vi "pcfs_auxillary_loop.vi"(8 "error in (no error)":errorcluster, 11 "pcfs in":refnum<class "pcfs.lvclass">) -> (0 "error out":errorcluster, 3 "pcfs out":refnum<class "pcfs.lvclass">)   [LabVIEW 2015, in "pcfs.lvclass"]
uses:
  pcfs.lvclass
  pcfs.lvclass/pcfs.ctl
  Detector_Class/Picoquant/Picoquant_generic/picoquant_generic.lvclass
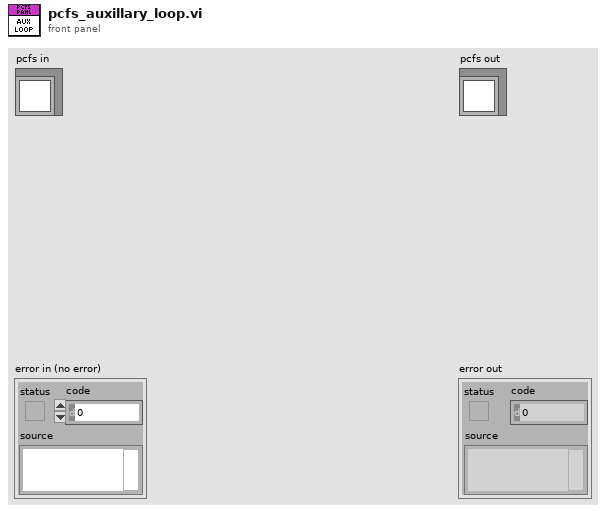
[diagram p1: front panel]
types:
  T1 = typedef "hydraharp_count_rates.ctl" = cluster{"channel_rates":i32[], "sync_rate":i32}
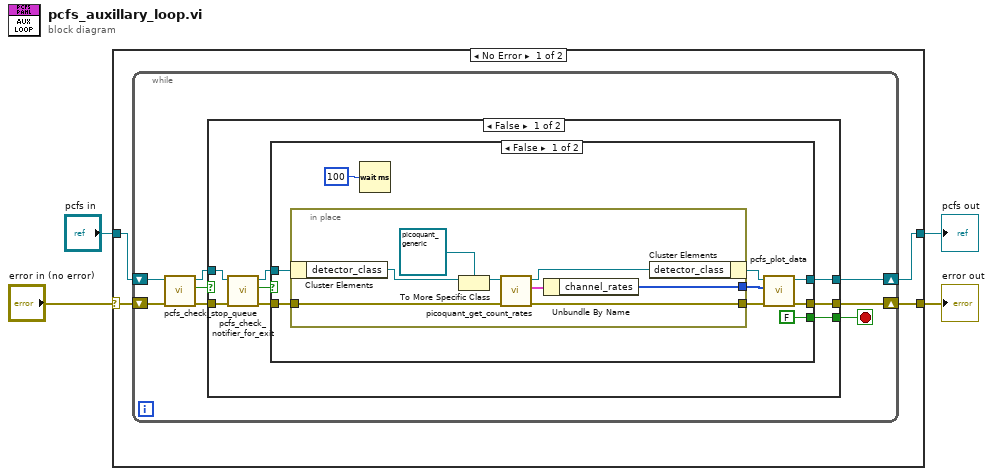
[diagram p0: block diagram]
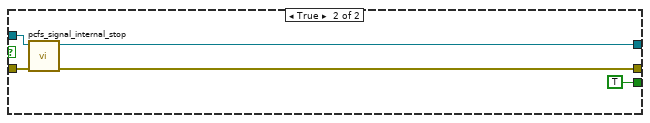
[diagram p3: hidden frame]
diagram:
  n1 = case shown="No Error" "error in (no error)" {
    selector: "error in (no error)" -> [w8 w51]
    tunnel: [w5 w51] -> w3
    tunnel: [w6 w50] -> w1
    tunnel: "pcfs in" -> [w7 w50]
    frame No Error {
      n2 = while {
        shift-right: [w15] -> w6
        shift-left: w7 -> [w12]
        shift-right: [w14] -> w5
        shift-left: w8 -> [w13]
        stop <- w16 stop-if-true
        n3 = call "pcfs_check_stop_queue.vi"("error in (no error)"=w13, "scan_panel in"=w12) -> ("error out"=w10:errorcluster, "stop?"=w9:bool, "scan_panel out"=w11:refnum<class "pcfs.lvclass">)  [unwired: 7 in]
        n4 = case shown="False" w9 {
          tunnel: [w23 TRUE] -> w16
          tunnel: [w20 w45] -> w15
          tunnel: [w19 w46] -> w14
          tunnel: w11 -> [w18 w49]
          tunnel: w10 -> [w17 w48]
          frame False {
            n5 = call "pcfs_check_notifier_for_exit.vi"("error in (no error)"=w17, "pcfs in"=w18) -> ("error out"=w22:errorcluster, "exit?"=w24:bool, "pcfs out"=w21:refnum<class "pcfs.lvclass">)  [unwired: 7 in]
            n6 = case shown="False" w24 {
              selector: w24 -> [_ w44]
              tunnel: [FALSE w44] -> w23
              tunnel: w22 -> [w31 w42]
              tunnel: w21 -> [w32 w43]
              tunnel: [w29 w43] -> w20
              tunnel: [w25 w42] -> w19
              frame False {
                n7 = in-place {
                  in-place-border: w31 -> [w38]
                  in-place-border: [w37] -> w28
                  in-place-border: [w34] -> w27
                  n8 = in-place-cluster #1(w32) -> ("detector_class"=w41:refnum<class "detector.lvclass">)
                  n9 = To More Specific Class(target class=refnum<class "picoquant_generic.lvclass"> refnum ("picoquant_generic in"), reference=w41) -> (specific class reference=w39:refnum<class "picoquant_generic.lvclass">)  [unwired: 1 in, 1 out]
                  n10 = call-dynamic "picoquant_get_count_rates.vi"("error in (no error)"=w38, "picoquant_generic in"=w39) -> ("error out"=w37:errorcluster, "count_rates"=w35:T1, "picoquant_generic out"=w36:refnum<class "picoquant_generic.lvclass">)  [unwired: 7 in]
                  n11 = Unbundle By Name(w35) -> ("channel_rates"=w34:i32[])
                  n12 = in-place-cluster #1("detector_class"=w36) -> (w30:refnum<class "pcfs.lvclass">)
                }
                n13 = Wait (ms)(milliseconds to wait=u32 100) -> ()  [unwired: 1 out]
                n14 = call "pcfs_plot_data.vi"("error in (no error)"=w28, "data"=w27, "scan_panel in"=w30) -> ("error out"=w25:errorcluster, "scan_panel out"=w29:refnum<class "pcfs.lvclass">)  [unwired: 7 in]
              }
              frame True {
              }
            }
          }
          frame True {
            n15 = call "pcfs_signal_internal_stop.vi"("error in (no error)"=w48, "pcfs in"=w49) -> ("error out"=w46:errorcluster, "pcfs out"=w45:refnum<class "pcfs.lvclass">)  [unwired: 8 in]
          }
        }
      }
    }
    frame Error {
    }
  }
  "error out" <- w3
  "pcfs out" <- w1
